vi "WalkWaypoint2.vi"(1 "check_block_size/2":i32, 2 "movement_limit":i32, 3 "Image Pixels (U8)":u8[][](array[numeric])) -> (0 "WaypointOut":cluster{i32, i32})   [LabVIEW 2009]
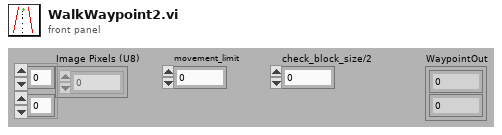
[diagram p1: front panel]
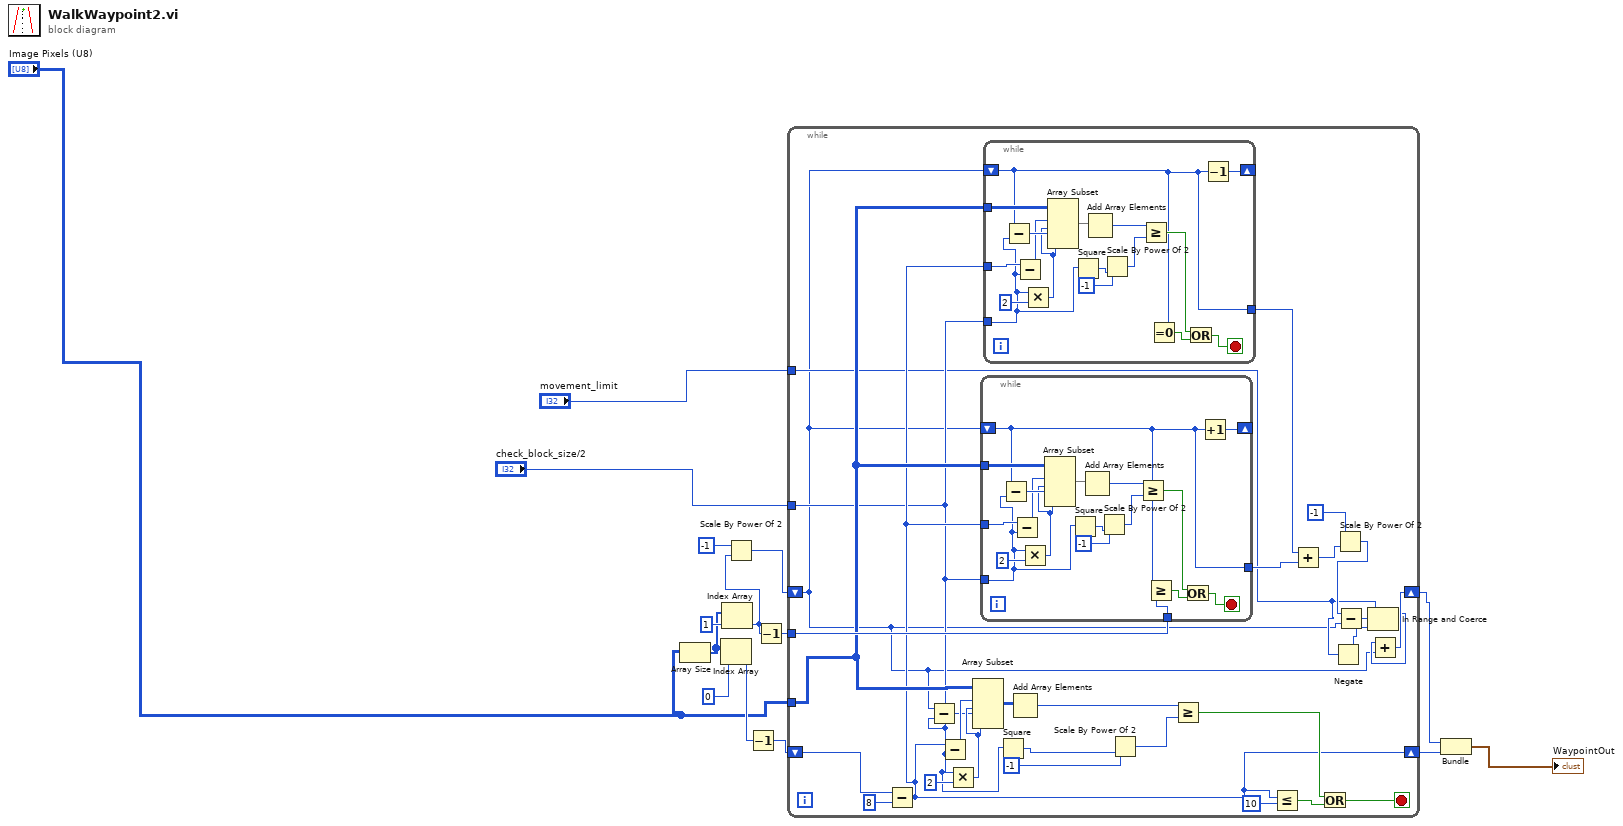
[diagram p0: block diagram]
diagram:
  n1 = Array Size(array="Image Pixels (U8)") -> (size(s)=w4:i32[])
  n2 = Index Array(array=w4, index=0) -> (element=w3:i32)
  n3 = Index Array(array=w4, index=1) -> (element=w8:i32)
  n4 = Scale By Power Of 2(n=-1, x=w8) -> (x*2^n=w7:i32)
  n5 = Decrement(x=w3) -> (x-1=w10:i32)
  n6 = Decrement(x=w8) -> (x-1=w9:i32)
  n7 = while {
    tunnel: "Image Pixels (U8)" -> [w23]
    shift-right: [w38] -> w14
    shift-left: w7 -> [w16]
    tunnel: w9 -> [w43]
    shift-right: [w21] -> w15
    shift-left: w10 -> [w24]
    tunnel: "check_block_size/2" -> [w18]
    tunnel: "movement_limit" -> [w17]
    stop <- w44 stop-if-true
    n8 = Subtract(x=w24, y=8) -> (x-y=w21:i32)
    n9 = Subtract(x=w16, y=w18) -> (x-y=w30:i32)
    n10 = Subtract(x=w21, y=w18) -> (x-y=w34:i32)
    n11 = Multiply(x=w18, y=2) -> (x*y=w31:i32)
    n12 = Array Subset(array=w23, index (row)=w34, length (row)=w31, index (col)=w30, length (col)=w31) -> (w33:u8[][])
    n13 = while {
      shift-right: [w80] -> _
      shift-left: w16 -> [w66]
      tunnel: [w66] -> w41
      tunnel: w43 -> [w77]
      tunnel: w23 -> [w67]
      tunnel: w21 -> [w65]
      tunnel: w18 -> [w64]
      stop <- w79 stop-if-true
      n14 = Subtract(x=w66, y=w64) -> (x-y=w72:i32)
      n15 = Subtract(x=w65, y=w64) -> (x-y=w68:i32)
      n16 = Multiply(x=w64, y=2) -> (x*y=w71:i32)
      n17 = Array Subset(array=w67, index (row)=w68, length (row)=w71, index (col)=w72, length (col)=w71) -> (w69:u8[][])
      n18 = Square(x=w64) -> (x^2=w73:i32)
      n19 = Add Array Elements(numeric array=w69) -> (sum=w75:u8)
      n20 = Scale By Power Of 2(n=-1, x=w73) -> (x*2^n=w76:i32)
      n21 = Greater Or Equal?(x=w75, y=w76) -> (x >= y?=w63:bool)
      n22 = Greater Or Equal?(x=w66, y=w77) -> (x >= y?=w78:bool)
      n23 = Or(x=w63, y=w78) -> (x .or. y?=w79:bool)
      n24 = Increment(x=w66) -> (x+1=w80:i32)
    }
    n25 = while {
      shift-right: [w62] -> _
      shift-left: w16 -> [w46]
      tunnel: [w46] -> w22
      tunnel: w23 -> [w50]
      tunnel: w21 -> [w49]
      tunnel: w18 -> [w48]
      stop <- w61 stop-if-true
      n26 = Subtract(x=w46, y=w48) -> (x-y=w55:i32)
      n27 = Subtract(x=w49, y=w48) -> (x-y=w51:i32)
      n28 = Multiply(x=w48, y=2) -> (x*y=w54:i32)
      n29 = Array Subset(array=w50, index (row)=w51, length (row)=w54, index (col)=w55, length (col)=w54) -> (w52:u8[][])
      n30 = Square(x=w48) -> (x^2=w56:i32)
      n31 = Add Array Elements(numeric array=w52) -> (sum=w58:u8)
      n32 = Scale By Power Of 2(n=-1, x=w56) -> (x*2^n=w59:i32)
      n33 = Greater Or Equal?(x=w58, y=w59) -> (x >= y?=w47:bool)
      n34 = Equal To 0?(x=w46) -> (x = 0?=w60:bool)
      n35 = Or(x=w47, y=w60) -> (x .or. y?=w61:bool)
      n36 = Decrement(x=w46) -> (x-1=w62:i32)
    }
    n37 = Square(x=w18) -> (x^2=w29:i32)
    n38 = Add Array Elements(numeric array=w33) -> (sum=w27:u8)
    n39 = Scale By Power Of 2(n=-1, x=w29) -> (x*2^n=w26:i32)
    n40 = Greater Or Equal?(x=w27, y=w26) -> (x >= y?=w25:bool)
    n41 = Less Or Equal?(x=w21, y=10) -> (x <= y?=w45:bool)
    n42 = Add(x=w22, y=w41) -> (x+y=w40:i32)
    n43 = Or(x=w25, y=w45) -> (x .or. y?=w44:bool)
    n44 = Negate(x=w17) -> (-x=w35:i32)
    n45 = Scale By Power Of 2(n=-1, x=w40) -> (x*2^n=w39:i32)
    n46 = Subtract(x=w39, y=w16) -> (x-y=w37:i32)
    n47 = In Range and Coerce(upper limit=w17, x=w37, lower limit=w35) -> (coerced(x)=w36:i32)  [unwired: 1 out]
    n48 = Add(x=w36, y=w16) -> (x+y=w38:i32)
  }
  n49 = Bundle(w14, w15) -> (→"WaypointOut":cluster{i32, i32})  [unwired: 1 in]
